vi "test_GetArrayElements.vi"() -> ()   [LabVIEW 2013]
uses:
  source/TypeDescriptor/TypeDescriptor_GetType.vi
  source/TypeDescriptor/TypeDescriptor_GetName.vi
  source/TypeDescriptor/TypeDescriptor_GetPString.vi
  source/Conversions/Flattened nD-Array to Flattened 1D-Array.vi
  source/Variant/OpenVariant.lvlib
panel:
  in  "Which Test?":bool
  in  "dims 2":string="4"
  in  "dim name 2":string="myString.size"
  in  "Data from KV pairs 2":string[](array[string])=["text", "in", "the", "array", "of", "strings"]
  in  "Element Names from KVP 2":string[](array[string])=["myString.Element[0]", "myString.Element[1]", "myString.Element[2]", "myString.Element[3]", "myString.Element[4]", "myString.Element[5]"]
  in  "dims":string="2 3"
  in  "dim name":string="Refnum.size"
  out "any found?":bool
  out "all found?":bool
  out "Rebuilt Array":variant
  out "Verification of Elements":variant[](array[variant])
  in  "Element Names from KVP":string[](array[string])=["Refnum.Numeric[0]", "Refnum.Numeric[1]", "Refnum.Numeric[2]", "Refnum.Numeric[3]", "Refnum.Numeric[4]", "Refnum.Numeric[5]"]
  in  "Data from KV pairs":dbl[](array[numeric])=[2.0, 4.0, 6.0, 8.0, 10.0, 12.0]
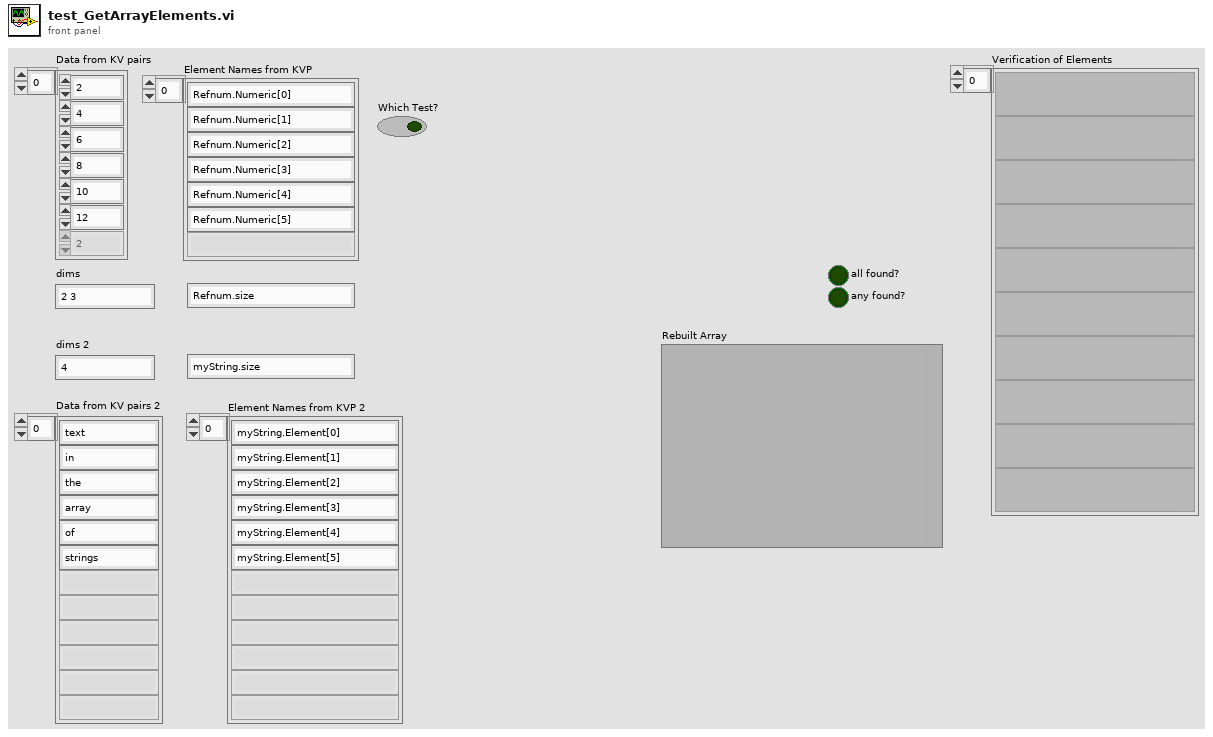
[diagram p1: front panel]
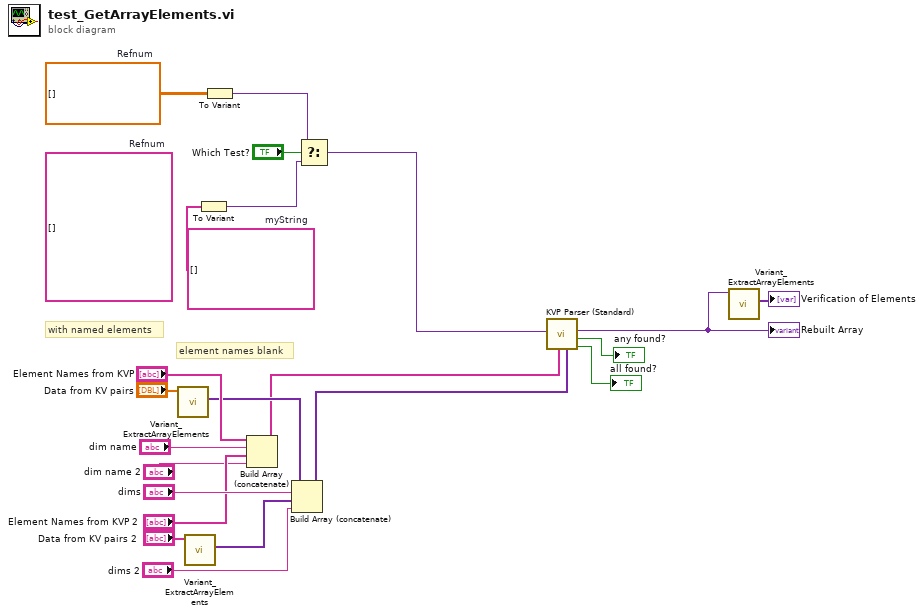
[diagram p0: block diagram]
diagram:
  w10 = string[] []  # myString
  (unwired) string[] []  # Refnum
  w21 = dbl[][] []  # Refnum
  # "element names blank"
  # "with named elements"
  n1 = call "Variant_ExtractArrayElements.vi"("Array"="Data from KV pairs") -> ("Elements"=w8:variant[])  [unwired: 7 in, 3 out]
  n2 = call "Variant_ExtractArrayElements.vi"("Array"="Data from KV pairs 2") -> ("Elements"=w7:variant[])  [unwired: 7 in, 3 out]
  n3 = To Variant(anything=w10) -> (Variant=w11:variant)
  n4 = To Variant(anything=w21) -> (Variant=w12:variant)
  n5 = Build Array (concatenate)("Element Names from KVP", "dim name", "Element Names from KVP 2", "dim name 2") -> (w5:string[])
  n6 = Build Array (concatenate)(w8, "dims", w7, "dims 2") -> (w4:variant[])
  n7 = Select(t=w12, s="Which Test?", f=w11) -> (s? t:f=w6:variant)
  n8 = call "KVP Parser (Standard).vi"("Values"=w4, "Keys"=w5, "Default Value"=w6) -> ("all found?"=→"all found?":bool, "any found?"=→"any found?":bool, "Value"=w3:variant)  [unwired: 5 in, 1 out]
  "Rebuilt Array" <- w3
  n9 = call "Variant_ExtractArrayElements.vi"("Array"=w3) -> ("Elements"=→"Verification of Elements":variant[])  [unwired: 7 in, 3 out]
